vi "RasterPI-Continuous1D.vi"(1 "Integration time":dbl, 2 "Step size":i32, 3 "Motor in":string, 4 "Steps":i32, 7 "Previous Speed":cluster{"VMIN":i32, "VMAX":i32, "ACC":i32}, 8 "Scan speed":cluster{"VMIN":i32, "VMAX":i32, "ACC":i32}, 9 "error in":errorcluster) -> (0 "Motor out":string, 5 "Graphe":dbl[](graph), 6 "error in (no error)":errorcluster caption="error out")   [LabVIEW 2009]
uses:
  Instruments/RTC/Api/TelemetryServer/TelemetryServer_Global.vi
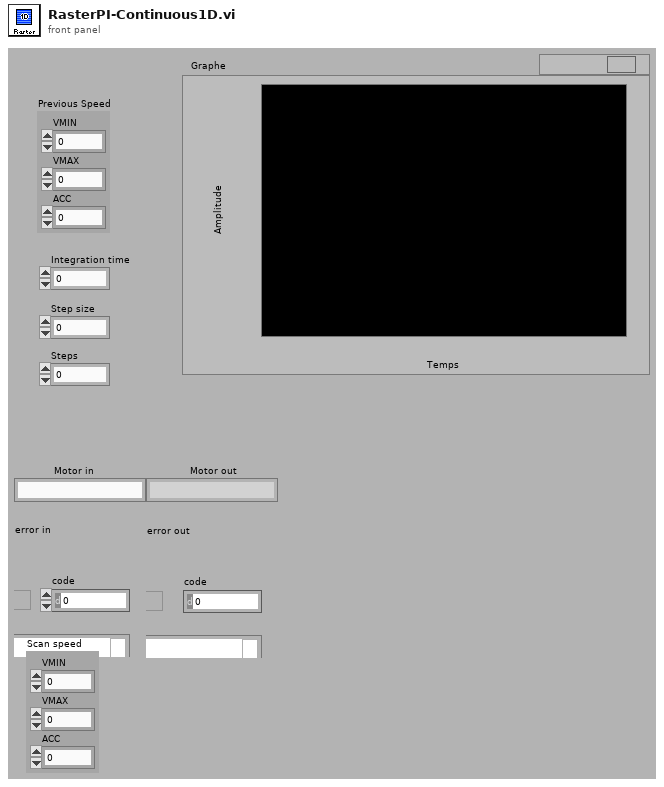
[diagram p1: front panel]
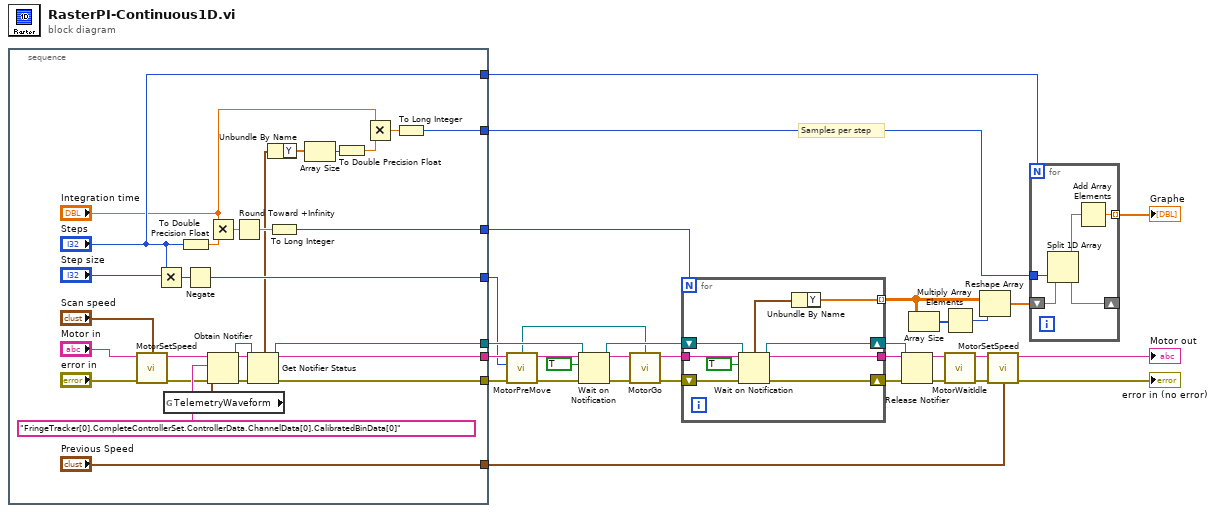
[diagram p0: block diagram]
diagram:
  # "Samples per step"
  n1 = stacked-sequence {
    tunnel: ["Previous Speed"] -> w29
    tunnel: [w52] -> w26
    tunnel: [w51] -> w19
    tunnel: [w50] -> w7
    tunnel: [w49] -> w13
    tunnel: [w45] -> w11
    tunnel: ["Steps"] -> w9
    tunnel: [w32] -> w8
    frame #0 {
      n2 = call "MotorSetSpeed.vi"("Param"="Scan speed", "Motor"="Motor in", "error in (no error)"="error in") -> ("Motor out"=w51:string, "error out"=w39:errorcluster)  [unwired: 5 out]
      n3 = Multiply(x="Step size", y="Steps") -> (x*y=w35:i32)
      n4 = global read "TelemetryServer_Global.vi" "TelemetryWaveform"() -> (w40:waveform(dbl))
      n5 = To Double Precision Float(number="Steps") -> (double precision float=w38:dbl)
      n6 = Negate(x=w35) -> (-x=w49:i32)
      n7 = Multiply(x="Integration time", y=w38) -> (x*y=w37:dbl)
      n8 = Obtain Notifier(name (unnamed)="FringeTracker[0].CompleteControllerSet.ControllerData.ChannelData[0].CalibratedBinData[0]" ("Telemetry"), notification data type=w40, error in (no error)=w39) -> (notifier out=w33:refnum<notifier>, error out=w34:errorcluster)  [unwired: 1 in, 1 out]
      n9 = Round Toward +Infinity(x=w37) -> (ceil(x): smallest int >= x=w36:dbl)
      n10 = Get Notifier Status(notifier=w33, error in (no error)=w34) -> (notifier out=w52:refnum<notifier>, current notification=w30:waveform(dbl), error out=w50:errorcluster)  [unwired: 2 out]
      n11 = Unbundle By Name(w30) -> ("Y"=w31:dbl[])
      n12 = To Long Integer(number=w36) -> (32bit integer=w32:i32)
      n13 = Array Size(array=w31) -> (size(s)=w48:i32)
      n14 = To Double Precision Float(number=w48) -> (double precision float=w47:dbl)
      n15 = Multiply(x="Integration time", y=w47) -> (x*y=w46:dbl)
      n16 = To Long Integer(number=w46) -> (32bit integer=w45:i32)
    }
  }
  n17 = call "MotorPreMove.vi"("Motor"=w19, "Movement"=w13, "error in (no error)"=w7) -> ("Motor out"=w5:string, "Go!"=w1:refnum<k4>, "error out"=w6:errorcluster)  [unwired: 4 out]
  n18 = Wait on Notification(notifier=w26, ignore previous (F)=TRUE ("ignorer précédent (F)"), error in (no error)=w6) -> (notifier out=w18:refnum<notifier>, error out=w4:errorcluster)  [unwired: 3 out]
  n19 = call "MotorGo.vi"("Go!"=w1, "Motor"=w5, "error in (no error)"=w4) -> ("Motor out"=w3:string, "error out"=w2:errorcluster)  [unwired: 5 out]
  n20 = for {
    N: w8 -> [_]
    shift-right: [w62] -> w24
    shift-left: w2 -> [w63]
    tunnel: w3 -> [w59]
    tunnel: [w57] -> w20 mode=indexing
    tunnel: [w59] -> w15
    shift-right: [w60] -> w23
    shift-left: w18 -> [w61]
    n21 = Wait on Notification(notifier=w61, ignore previous (F)=TRUE ("ignorer précédent (F)"), error in (no error)=w63) -> (notifier out=w60:refnum<notifier>, notification=w58:waveform(dbl), error out=w62:errorcluster)  [unwired: 2 out]
    n22 = Unbundle By Name(w58) -> ("Y"=w57:dbl[])
  }
  n23 = Release Notifier(notifier=w23, error in (no error)=w24) -> (error out=w17:errorcluster)  [unwired: 3 out]
  n24 = Array Size(array=w20) -> (size(s)=w22:i32[])
  n25 = Multiply Array Elements(1:w22) -> (0:w21:i32)
  n26 = call "MotorWaitIdle.vi"("Motor"=w15, "error in (no error)"=w17) -> ("Motor out"=w14:string, "error out"=w16:errorcluster)  [unwired: 6 out]
  n27 = Reshape Array(w20, w21) -> (w12:dbl[])
  n28 = call "MotorSetSpeed.vi"("Param"=w29, "Motor"=w14, "error in (no error)"=w16) -> ("Motor out"=→"Motor out":string, "error out"=→"error in (no error)":errorcluster)  [unwired: 5 out]
  n29 = for {
    N: w9 -> [_]
    shift-right: [w66] -> _
    shift-left: w12 -> [w68]
    tunnel: w11 -> [w69]
    tunnel: [w65] -> w10 mode=indexing
    n30 = Split 1D Array(array=w68, index=w69) -> (first subarray=w67:dbl[], second subarray=w66:dbl[])
    n31 = Add Array Elements(numeric array=w67) -> (sum=w65:dbl)
  }
  "Graphe" <- w10
